vi "Write All Data Words.vi"(6 "Data Words":u16[](array[numeric]), 8 "Error In":errorcluster, 9 "Buffer Type":T1(ring)=enum."BC Message Buffer", 10 "Buffer Header and Buffer ID":u16=1, 11 "Module Handle":u32) -> (0 "Error Out":errorcluster, 3 "Module Handle out":u32)   [LabVIEW 2020, in "AIM MIL-STD-1553 Hardware API.lvlib"]
uses:
  AIM MIL-STD-1553 Hardware API.lvlib
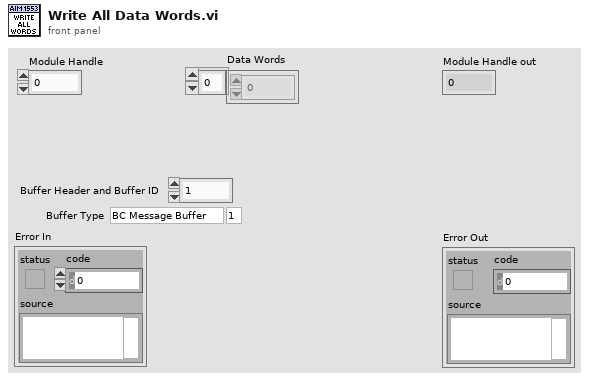
[diagram p1: front panel]
types:
  T1 = enum16{"unknown", "BC Message Buffer", "RT Message Buffer"}
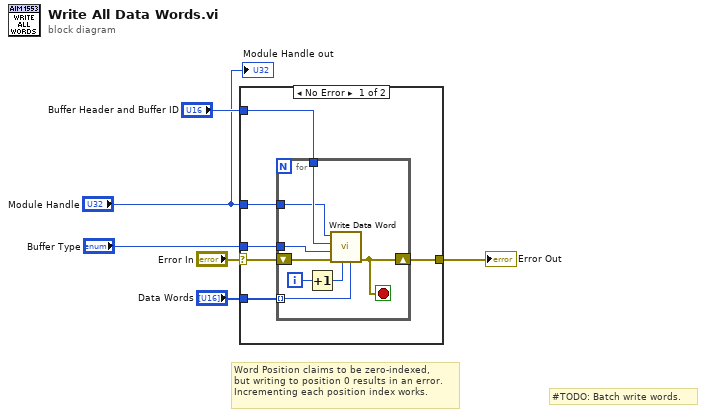
[diagram p0: block diagram]
diagram:
  # "#TODO: Batch write words."
  # "Word Position claims to be zero-indexed,\nbut writing to position 0 results in an error.\nIncrementing each position index works."
  n1 = case shown="No Error" "Error In" {
    selector: "Error In" -> [w12 w21]
    tunnel: [w9 w21] -> w6
    tunnel: "Buffer Type" -> [w11 _]
    tunnel: "Buffer Header and Buffer ID" -> [w10 _]
    tunnel: "Data Words" -> [w7 _]
    tunnel: "Module Handle" -> [w8 _]
    frame No Error {
      n2 = for {
        tunnel: w11 -> [w19]
        tunnel: w10 -> [w18]
        tunnel: w8 -> [w17]
        shift-right: [w14] -> w9
        shift-left: w12 -> [w20]
        tunnel: w7 -> [w16] mode=indexing
        i -> [w15]
        stop <- w14 stop-if-true
        n3 = Increment(x=w15) -> (x+1=w13:i32)
        n4 = call "Write Data Word.vi"("Data Word to Write"=w16, "Word Position"=w13, "Error In"=w20, "Buffer Type"=w19, "Buffer Header and Buffer ID"=w18, "Module Handle"=w17) -> ("Error Out"=w14:errorcluster)  [unwired: 4 in, 1 out]
      }
    }
    frame Error {
    }
  }
  "Error Out" <- w6
  "Module Handle out" <- "Module Handle"
